vi "Zip Output.vi"(8 "error in (no error)":errorcluster, 10 "Generated Files":path[](array[path]), 11 "Zip File Location":path) -> (0 "error out":errorcluster)   [LabVIEW 2014, in "G CLI LvBuild.lvlib"]
uses:
  G CLI LvBuild.lvlib
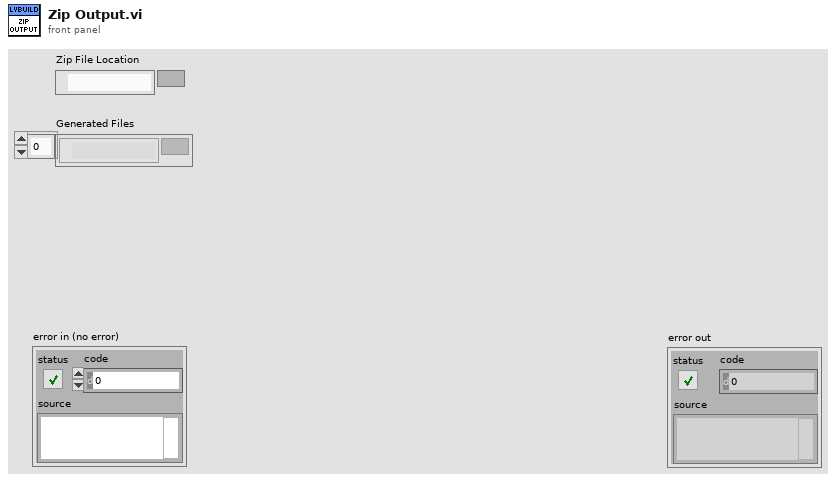
[diagram p1: front panel]
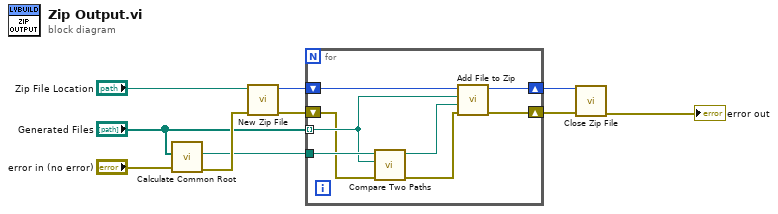
[diagram p0: block diagram]
diagram:
  n1 = call "Calculate Common Root.vi"("error in (no error)"="error in (no error)", "Generated Files"="Generated Files") -> ("error out"=w9:errorcluster, "Root Path"=w1:path)  [unwired: 8 in]
  n2 = call <vilib>:"New Zip File.vi"("error in (no error)"=w9, "target"="Zip File Location") -> ("error out"=w7:errorcluster, "zip file out"=w5:i64)  [unwired: 3 in, 1 out]
  n3 = for {
    shift-right: [w18] -> w6
    shift-left: w7 -> [w13]
    shift-right: [w16] -> w4
    shift-left: w5 -> [w17]
    tunnel: "Generated Files" -> [w14] mode=indexing
    tunnel: w1 -> [w15]
    n4 = call <vilib>:"Compare Two Paths.vi"("error in (no error)"=w13, "Path 2"=w14, "Path 1"=w15) -> ("error out"=w12:errorcluster, "Relative Path from 1 to 2"=w11:path)  [unwired: 5 in, 2 out]
    n5 = call <vilib>:"Add File to Zip.vi"("error in (no error)"=w12, "destination path in zip"=w11, "source file path"=w14, "zip file in"=w17) -> ("error out"=w18:errorcluster, "zip file out"=w16:i64)  [unwired: 6 in]
  }
  n6 = call <vilib>:"Close Zip File.vi"("error in (no error)"=w6, "zip file in"=w4) -> ("error out"=→"error out":errorcluster)  [unwired: 5 in]
